vi "Plot Record.vi"() -> ()   [LabVIEW 2015]
uses:
  <vilib>/Utility/file.llb/Read From Spreadsheet File (I64).vi
panel:
  in  "Start position":i32 format="%.0p"
  out "Array size":i32
  in  "Max Volts":dbl=1.0
  in  "Read samples":i32=-1 format="%.0p"
  in  "ASCII?":bool
  out "Waveform Graph":cluster{dbl, dbl, "Volts":dbl[]}(graph)
  in  "Save to File":path=path "D:/Data/dump.bin"
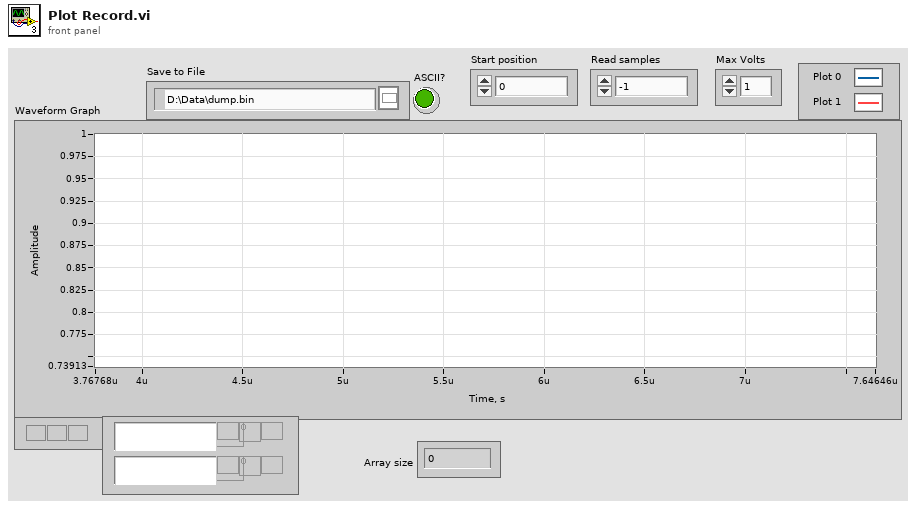
[diagram p1: front panel]
types:
  T1 = enum16{"big-endian, network order", "native, host order", "little-endian"}
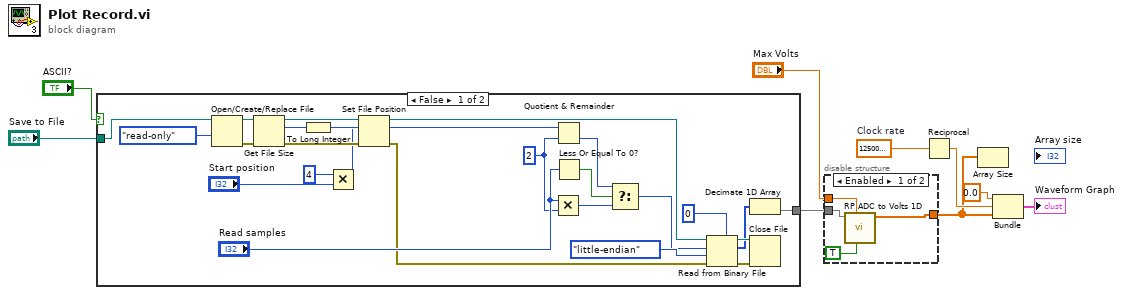
[diagram p0: block diagram]
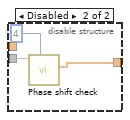
[diagram p2: hidden frame]
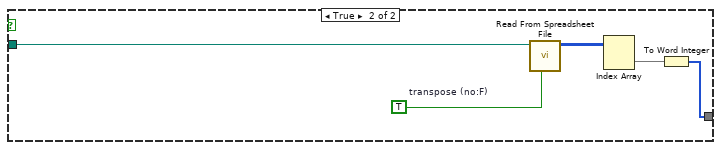
[diagram p3: hidden frame]
diagram:
  w3 = 125000000.0  # Clock rate
  n1 = case shown="False" "ASCII?" {
    tunnel: "Save to File" -> [w34 w39]
    tunnel: [w16 w36] -> w8
    frame False {
      w17 = 2 ("y")
      n2 = Open/Create/Replace File(file path (use dialog)=w34, access (0:read/write)=enum16{"read/write", "read-only", "write-only"}."read-only") -> (refnum out=w28:refnum<file>, error out=w29:errorcluster)  [unwired: 4 in, 1 out]
      n3 = Get File Size(file=w28, error in=w29) -> (refnum out=w27:refnum<file>, size (in bytes)=w26:i64, 0:w13:errorcluster)
      n4 = To Long Integer(number=w26) -> (32bit integer=w22:i32)
      n5 = Multiply(x=4, y="Start position") -> (x*y=w11:i32)
      n6 = Set File Position(offset (in bytes) (0)=w11, refnum=w27, error in=w13) -> (refnum out=w15:refnum<file>, error out=w12:errorcluster)  [unwired: 1 in]
      n7 = Multiply(x="Read samples", y=w17) -> (x*y=w19:i32)
      n8 = Quotient & Remainder(x=w22, y=w17) -> (floor(x/y)=w20:i32)  [unwired: 1 out]
      n9 = Less Or Equal To 0?(x="Read samples") -> (x <= 0?=w23:bool)
      n10 = Select(t=w20, s=w23, f=w19) -> (s? t:f=w21:i32)
      n11 = Read from Binary File(5:i16 0, 8:w12, 9:T1."little-endian" ("byte order (0:big-endian, network order)"), 10:w21, 11:w15) -> (0:w31:errorcluster, 2:w25:i16[], 3:w32:refnum<file>)  [unwired: 1 in, 1 out]
      n12 = Decimate 1D Array(w25) -> (w16:i16[])  [unwired: 1 out]
      n13 = Close File(refnum=w32, error in=w31) -> ()  [unwired: 2 out]
    }
    frame True {
      w37 = TRUE  # transpose (no:F)
      n14 = call-poly <vilib>:"Read From Spreadsheet File.vi"("transpose (no:F)"=w37, "file path (dialog if empty)"=w39) -> ("all rows"=w38:i64[][])  [unwired: 5 in, 4 out]
      n15 = Index Array(array=w38) -> (element=w35:i64[])  [unwired: 2 in]
      n16 = To Word Integer(number=w35) -> (16bit integer=w36:i16[])
    }
  }
  n17 = disable-structure shown="Enabled" {
    disable-tunnel: w8 -> [w43 w46]
    disable-tunnel: [w42 w44] -> w1
    disable-tunnel: "Max Volts" -> [w41 _]
    frame Enabled {
      n18 = call "RP ADC to Volts 1D.vi"("osc_fpga_cnv_cnt_to_v method"=TRUE, "Max Volts"=w41, "ADC data"=w43) -> ("Volts"=w42:dbl[])  [unwired: 8 in]
    }
    frame Disabled {
      n19 = call "Phase shift check.vi"("Half period"=4, "Wave form"=w46) -> ("theta"=w44:dbl[])  [unwired: 8 in, 1 out]
    }
  }
  n20 = Reciprocal(x=w3) -> (1/x=w2:dbl)
  n21 = Array Size(array=w1) -> ()  [unwired: 1 out]
  n22 = Bundle(0.0, w2, "Volts"=w1) -> (→"Waveform Graph":cluster{dbl, dbl, "Volts":dbl[]})  [unwired: 1 in]
